vi "replayReplace.vi"(0 "Game in":refnum<class "Game.lvclass">, 1 "On":bool, 2 "vision?":bool=TRUE, 3 "unsigned byte array":u8[](array[numeric]), 4 "Play":bool, 5 "error in (no error)":errorcluster, 7 "Enable":bool, 13 "Slide":dbl(slide) scale=0.0..10.0) -> (14 "Game out":refnum<class "Game.lvclass">, 15 "delay":dbl, 16 "ReplayInfo":T1, 17 "unsigned byte array out":u8[](array[numeric]), 18 "Slide out":dbl(slide) scale=0.0..10.0, 19 "error out":errorcluster)   [LabVIEW 2020, in "Game.lvclass"]
uses:
  Game.lvclass
  ReplayInfo.ctl
  RobotExtraInfo.ctl
  Utilities_class/Utilities.lvclass
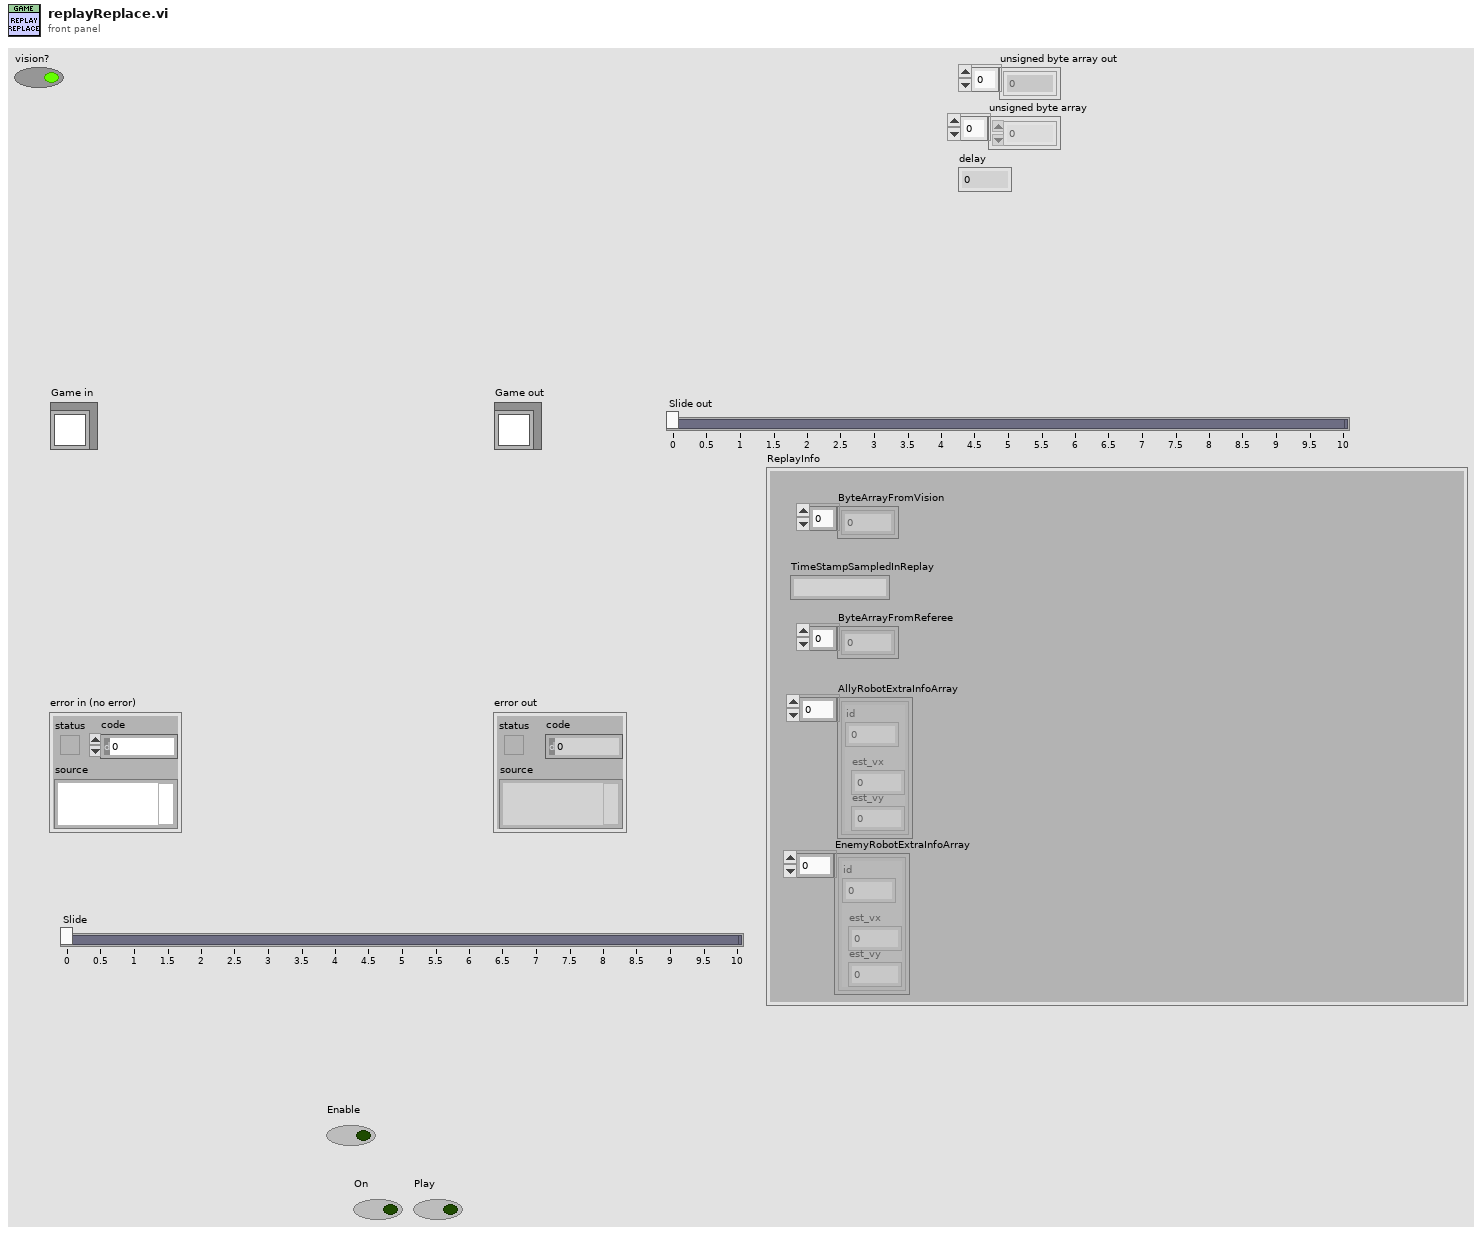
[diagram p1: front panel]
types:
  T1 = typedef "ReplayInfo.ctl" = cluster{"ByteArrayFromVision":u8[], "TimeStampSampledInReplay":string, "ByteArrayFromReferee":u8[], "AllyRobotExtraInfoArray":T2[], "EnemyRobotExtraInfoArray":T2[]}
  T2 = typedef "RobotExtraInfo.ctl" = cluster{"est_vx":dbl, "est_vy":dbl, "id":dbl}
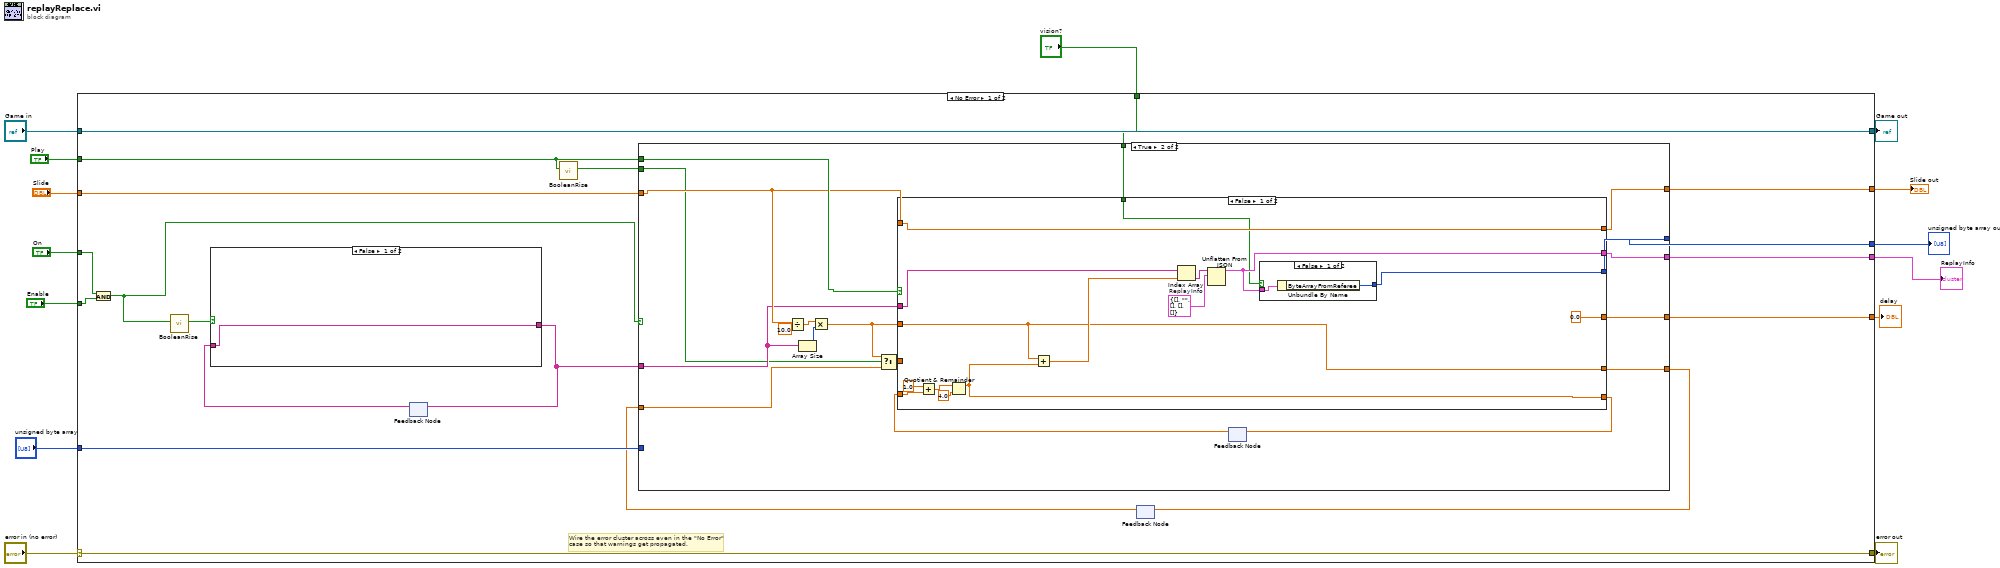
[diagram p0: block diagram]
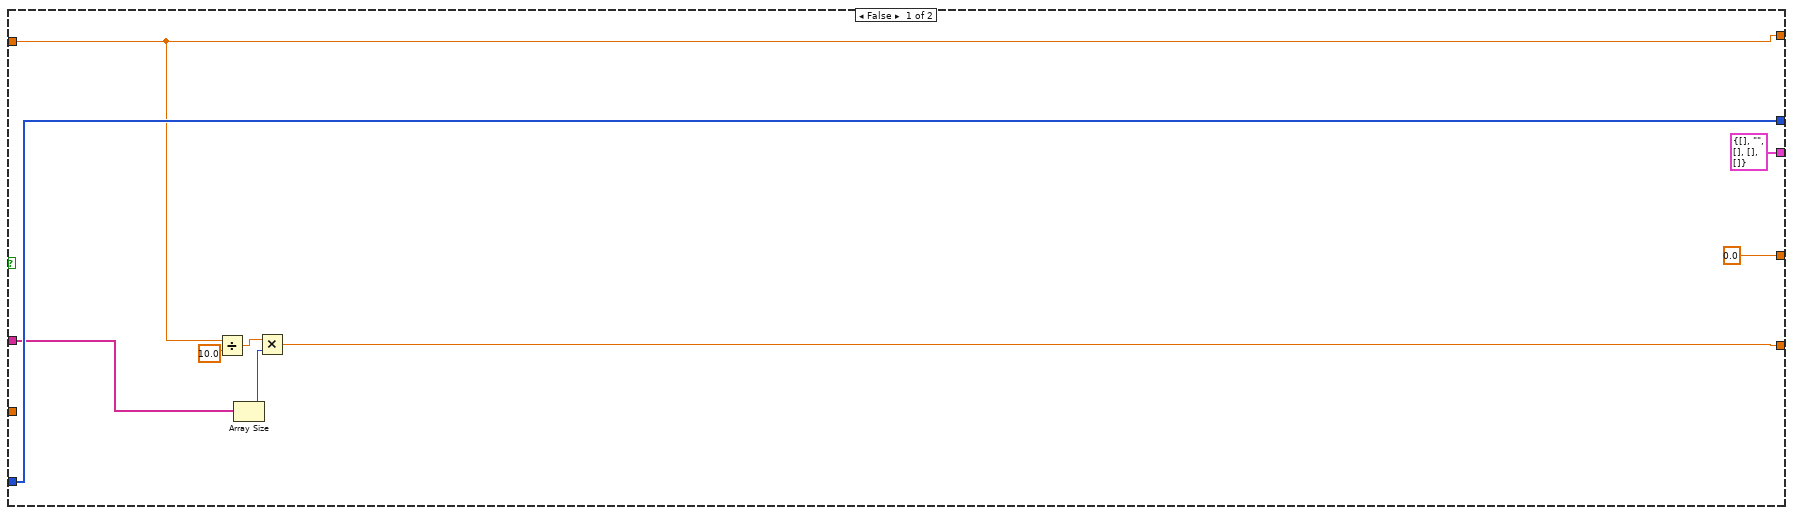
[diagram p2: hidden frame]
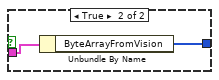
[diagram p3: hidden frame]
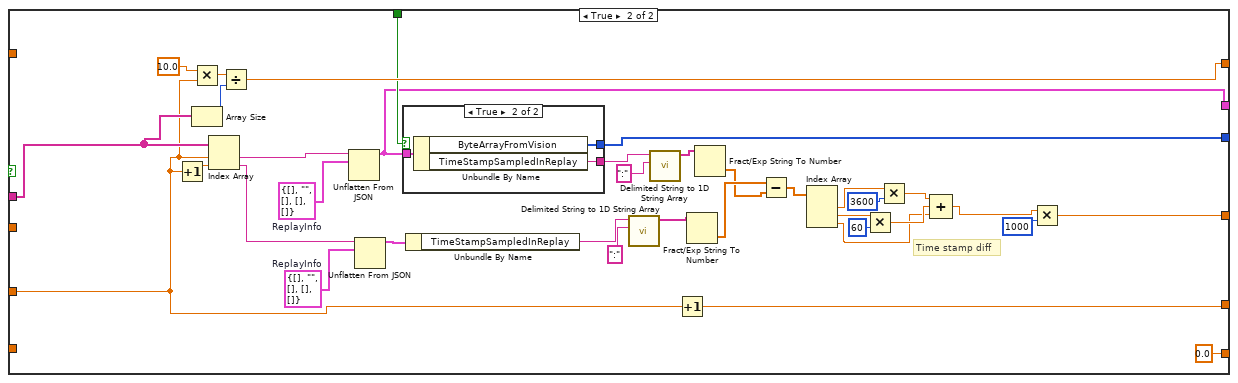
[diagram p4: hidden frame]
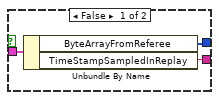
[diagram p5: hidden frame]
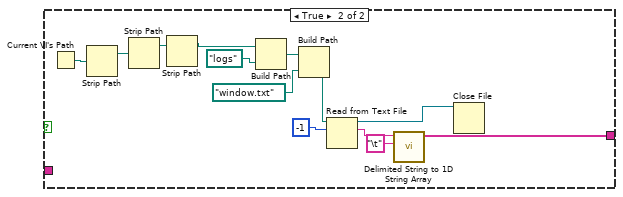
[diagram p6: hidden frame]
diagram:
  n1 = case shown="No Error" "error in (no error)" {
    selector: "error in (no error)" -> [w32 w137]
    tunnel: [w32 w137] -> w13
    tunnel: [w33 w136] -> w11
    tunnel: "Game in" -> [w33 w136]
    tunnel: "Enable" -> [w30 _]
    tunnel: "Play" -> [w18 _]
    tunnel: "On" -> [w20 _]
    tunnel: "Slide" -> [w31 _]
    tunnel: [w29 _] -> w2
    tunnel: "unsigned byte array" -> [w28 _]
    tunnel: [w27 _] -> w5
    tunnel: [w26 _] -> w4
    tunnel: "vision?" -> [w25 _]
    tunnel: [w24 _] -> w1
    frame No Error {
      # "Wire the error cluster across even in the \"No Error\"\ncase so that warnings get propagated."
      n2 = And(x=w20, y=w30) -> (x .and. y?=w23:bool)
      n3 = call "BooleanRise.vi"("Boolean in"=w23) -> ("Boolean"=w21:bool)  [unwired: 8 in, 2 out]
      n4 = feedback #1() -> (w22:string[])  [unwired: 1 in]
      n5 = case shown="False" w21 {
        tunnel: [w122 w132] -> w15
        tunnel: w22 -> [w122 _]
        frame False {
        }
        frame True {
          n6 = Current VI's Path() -> (path=w128:path)
          n7 = Strip Path(path=w128) -> (stripped path=w129:path)  [unwired: 1 out]
          n8 = Strip Path(path=w129) -> (stripped path=w124:path)  [unwired: 1 out]
          n9 = Strip Path(path=w124) -> (stripped path=w123:path)  [unwired: 1 out]
          n10 = Build Path(base path=w123, name or relative path=path "logs") -> (appended path=w130:path)
          n11 = Build Path(base path=w130, name or relative path=path "window.txt") -> (appended path=w125:path)
          n12 = Read from Text File(file (use dialog)=w125, count=-1) -> (refnum out=w131:refnum<file>, text=w134:string)  [unwired: 2 in, 2 out]
          n13 = call <vilib>:"Delimited String to 1D String Array.vi"("delimiter"="\t", "delimited string"=w134) -> ("string array"=w132:string[])  [unwired: 9 in]
          n14 = Close File(refnum=w131) -> ()  [unwired: 1 in, 2 out]
        }
      }
      n15 = feedback-in #1(w15) -> ()
      n16 = call "BooleanRise.vi"("Boolean in"=w18) -> ("Boolean"=w19:bool)  [unwired: 8 in, 2 out]
      n17 = feedback #2() -> (w16:dbl)  [unwired: 1 in]
      n18 = case shown="True" w23 {
        tunnel: w31 -> [w35 w58]
        tunnel: [w42 w60] -> w29
        tunnel: w28 -> [w42 _]
        tunnel: w18 -> [_ w59]
        tunnel: [w35 w54] -> w27
        tunnel: [0.0 w53] -> w26
        tunnel: w25 -> [_ w52]
        tunnel: [T1 {"ByteArrayFromVision"=[], "TimeStampSampledInReplay"="", "ByteArrayFromReferee"=[], "AllyRobotExtraInfoArray"=[], "EnemyRobotExtraInfoArray"=[]} ("ReplayInfo") w51] -> w24
        tunnel: w15 -> [w36 w50]
        tunnel: w19 -> [_ w48]
        tunnel: [w34 w46] -> w17
        tunnel: w16 -> [_ w45]
        frame False {
          n19 = Divide(x=w35, y=10.0) -> (x/y=w38:dbl)
          n20 = Array Size(array=w36) -> (size(s)=w37:i32)
          n21 = Multiply(x=w38, y=w37) -> (x*y=w34:dbl)
        }
        frame True {
          n22 = Divide(x=w58, y=10.0) -> (x/y=w56:dbl)
          n23 = Array Size(array=w50) -> (size(s)=w55:i32)
          n24 = Multiply(x=w56, y=w55) -> (x*y=w49:dbl)
          n25 = Select(t=w49, s=w48, f=w45) -> (s? t:f=w47:dbl)
          n26 = feedback #3() -> (w43:dbl)  [unwired: 1 in]
          n27 = case shown="False" w59 {
            tunnel: w58 -> [w72 _]
            tunnel: w50 -> [w75 w97]
            tunnel: [w68 w100] -> w60
            tunnel: [w72 w96] -> w54
            tunnel: [w66 w86] -> w46
            tunnel: w47 -> [_ w90]
            tunnel: w49 -> [w66 _]
            tunnel: [0.0 w83] -> w53
            tunnel: w52 -> [w69 w82]
            tunnel: [w70 w81] -> w51
            tunnel: [w61 0.0] -> w44
            tunnel: w43 -> [w65 _]
            frame False {
              w73 = T1 {"ByteArrayFromVision"=[], "TimeStampSampledInReplay"="", "ByteArrayFromReferee"=[], "AllyRobotExtraInfoArray"=[], "EnemyRobotExtraInfoArray"=[]}  # ReplayInfo
              n28 = Add(x=1.0, y=w65) -> (x+y=w63:dbl)
              n29 = Quotient & Remainder(x=w63, y=4.0) -> (x-y*floor(x/y)=w61:dbl)  [unwired: 1 out]
              n30 = Add(x=w66, y=w61) -> (x+y=w67:dbl)
              n31 = Index Array(array=w75, index=w67) -> (element=w74:string)
              n32 = Unflatten From JSON(JSON string=w74, type and defaults=w73) -> (value=w70:T1)  [unwired: 5 in, 1 out]
              n33 = case shown="False" w69 {
                tunnel: w70 -> [w77 w79]
                tunnel: [w76 w78] -> w68
                frame False {
                  n34 = Unbundle By Name(w77) -> ("ByteArrayFromReferee"=w76:u8[])
                }
                frame True {
                  n35 = Unbundle By Name(w79) -> ("ByteArrayFromVision"=w78:u8[])
                }
              }
            }
            frame True {
              w113 = T1 {"ByteArrayFromVision"=[], "TimeStampSampledInReplay"="", "ByteArrayFromReferee"=[], "AllyRobotExtraInfoArray"=[], "EnemyRobotExtraInfoArray"=[]}  # ReplayInfo
              w115 = T1 {"ByteArrayFromVision"=[], "TimeStampSampledInReplay"="", "ByteArrayFromReferee"=[], "AllyRobotExtraInfoArray"=[], "EnemyRobotExtraInfoArray"=[]}  # ReplayInfo
              # "Time stamp diff"
              n36 = Increment(x=w90) -> (x+1=w114:dbl)
              n37 = Multiply(x=10.0 ("y"), y=w90) -> (x*y=w99:dbl)
              n38 = Array Size(array=w97) -> (size(s)=w98:i32)
              n39 = Index Array(array=w97, index #1=w90, index #2=w114) -> (element #1=w112:string, element #2=w87:string)
              n40 = Divide(x=w99, y=w98) -> (x/y=w96:dbl)
              n41 = Unflatten From JSON(JSON string=w112, type and defaults=w115) -> (value=w81:T1)  [unwired: 5 in, 1 out]
              n42 = Unflatten From JSON(JSON string=w87, type and defaults=w113) -> (value=w111:T1)  [unwired: 5 in, 1 out]
              n43 = case shown="True" w82 {
                tunnel: w81 -> [w118 w121]
                tunnel: [w116 w120] -> w100
                tunnel: [w117 w119] -> w92
                frame False {
                  n44 = Unbundle By Name(w118) -> ("ByteArrayFromReferee"=w116:u8[], "TimeStampSampledInReplay"=w117:string)
                }
                frame True {
                  n45 = Unbundle By Name(w121) -> ("ByteArrayFromVision"=w120:u8[], "TimeStampSampledInReplay"=w119:string)
                }
              }
              n46 = Unbundle By Name(w111) -> ("TimeStampSampledInReplay"=w94:string)
              n47 = call <vilib>:"Delimited String to 1D String Array.vi"("delimiter"=":" ("delimited string"), "delimited string"=w94) -> ("string array"=w89:string[])  [unwired: 9 in]
              n48 = call <vilib>:"Delimited String to 1D String Array.vi"("delimiter"=":" ("delimited string"), "delimited string"=w92) -> ("string array"=w88:string[])  [unwired: 9 in]
              n49 = Increment(x=w90) -> (x+1=w86:dbl)
              n50 = Fract/Exp String To Number(string=w89) -> (number=w85:dbl[])  [unwired: 3 in, 1 out]
              n51 = Fract/Exp String To Number(string=w88) -> (number=w84:dbl[])  [unwired: 3 in, 1 out]
              n52 = Subtract(x=w85, y=w84) -> (x-y=w110:dbl[])
              n53 = Index Array(array=w110) -> (element #1=w109:dbl, element #2=w108:dbl, element #3=w103:dbl)  [unwired: 3 in]
              n54 = Multiply(x=w108, y=60) -> (x*y=w104:dbl)
              n55 = Multiply(x=w109, y=3600) -> (x*y=w105:dbl)
              n56 = Compound Arithmetic op=ADD(w105, w104, w103) -> (w102:dbl)
              n57 = Multiply(x=w102, y=1000) -> (x*y=w83:dbl)
            }
          }
          n58 = feedback-in #3(w44) -> ()
        }
      }
      n59 = feedback-in #2(w17) -> ()
    }
    frame Error {
    }
  }
  "error out" <- w13
  "Game out" <- w11
  "Slide out" <- w5
  "unsigned byte array out" <- w2
  "delay" <- w4
  "ReplayInfo" <- w1
